vi "log data.vi"(5 "power monitor queue in":refnum<queue>, 7 "i2c queue in":refnum<queue>, 8 "error in":errorcluster, 9 "path":string, 10 "register monitor queue in":refnum<queue>, 11 "image queue in":refnum<queue>) -> (0 "error out":errorcluster)   [LabVIEW 2025, in "Automotive Vision.lvclass"]
uses:
  Automotive Vision.lvclass
  Automotive Vision.lvclass/Automotive Vision.ctl
  regitster_value.ctl
  power.ctl
  image.ctl
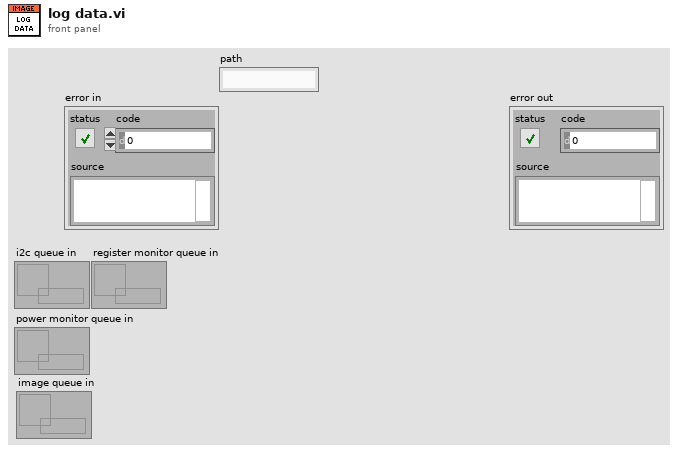
[diagram p1: front panel]
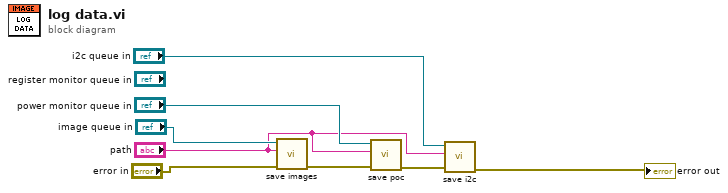
[diagram p0: block diagram]
diagram:
  n1 = call "save images.vi"("error in"="error in", "path"="path", "image queue in"="image queue in") -> ("error out"=w6:errorcluster)  [unwired: 8 in]
  n2 = call "save poc.vi"("error in"=w6, "path"="path", "power monitor queue in"="power monitor queue in") -> ("error out"=w4:errorcluster)  [unwired: 8 in]
  n3 = call "save i2c.vi"("error in"=w4, "path"="path", "i2c queue in"="i2c queue in") -> ("error out"=→"error out":errorcluster)  [unwired: 8 in]
